vi "RS_ext.vi"(2 "Q old":bool, 3 "R":bool, 4 "S":bool) -> (0 "~Q":bool=TRUE, 1 "Q":bool)   [LabVIEW 2019, in "Triggers.lvlib"]
uses:
  Triggers.lvlib
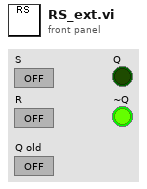
[diagram p1: front panel]
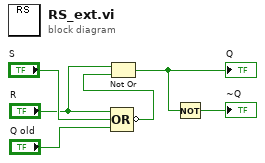
[diagram p0: block diagram]
diagram:
  n1 = Compound Arithmetic op=OR("R", "S", "Q old") -> (invert w6:bool)
  n2 = Not Or(1:w6, 2:"R") -> (0:w4:bool)
  "Q" <- w4
  n3 = Not(x=w4) -> (.not. x?=→"~Q":bool)
